vi "Write to Digital Line.vi"() -> ()   [LabVIEW 2020]
uses:
  <vilib>/DAQmx/write.llb/DAQmx Write (Digital Bool 1Line 1Point).vi
  <vilib>/DAQmx/create/channels.llb/DAQmx Create Channel (DO-Digital Output).vi
  <vilib>/DAQmx/miscellaneous.llb/DAQmx Fill In Error Info.vi
panel:
  in  "stop":bool
  in  "Boolean":bool
  in  "DAQmx Physical Channel":tag
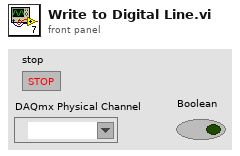
[diagram p1: front panel]
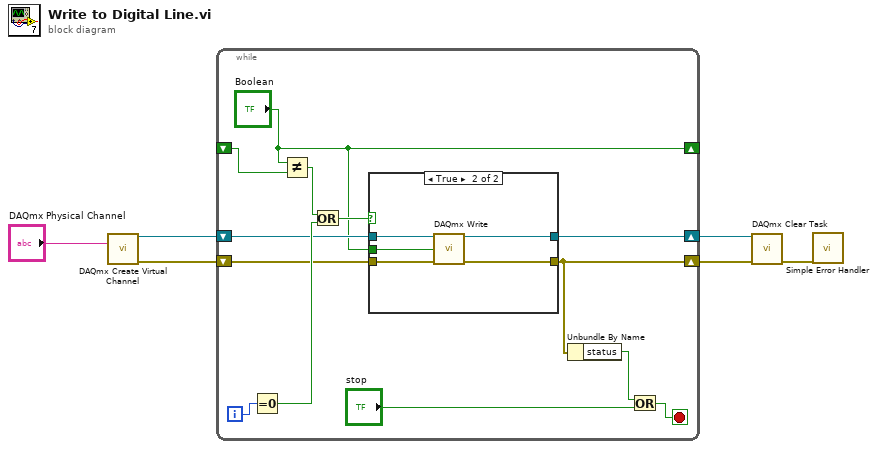
[diagram p0: block diagram]
diagram:
  n1 = call-poly <vilib>:"DAQmx Create Virtual Channel.vi"("lines"="DAQmx Physical Channel") -> ("task out"=w5:refnum<k21>, "error out"=w4:errorcluster)  [unwired: 13 in]
  n2 = while {
    shift-right: ["Boolean"] -> _
    shift-left: _ -> [w18]
    shift-right: [w8] -> w2
    shift-left: w4 -> [w13]
    shift-right: [w11] -> w3
    shift-left: w5 -> [w14]
    i -> [w19]
    stop <- w10 stop-if-true
    n3 = Equal To 0?(x=w19) -> (x = 0?=w16:bool)
    n4 = Not Equal?(x="Boolean", y=w18) -> (x != y?=w17:bool)
    n5 = Or(x=w17, y=w16) -> (x .or. y?=w15:bool)
    n6 = case shown="True" w15 {
      tunnel: w14 -> [w21 w26]
      tunnel: w13 -> [w20 w25]
      tunnel: "Boolean" -> [_ w24]
      tunnel: [w21 w23] -> w11
      tunnel: [w20 w22] -> w8
      frame False {
      }
      frame True {
        n7 = call-poly <vilib>:"DAQmx Write.vi"("task/channels in"=w26, "data"=w24, "error in"=w25) -> ("task out"=w23:refnum<k21>, "error out"=w22:errorcluster)  [unwired: 10 in, 1 out]
      }
    }
    n8 = Unbundle By Name "Unbundle By Name"(w8) -> ("status"=w7:bool)
    n9 = Or(x=w7, y="stop") -> (x .or. y?=w10:bool)
  }
  n10 = call <vilib>:"DAQmx Clear Task.vi"("task in"=w3, "error in"=w2) -> ("error out"=w1:errorcluster)  [unwired: 13 in]
  n11 = call <vilib>:"Simple Error Handler.vi"("error in (no error)"=w1) -> ()  [unwired: 4 in, 5 out]
